vi "Check Configs Exist.vi"(8 "error in (no error)":errorcluster, 11 "picoG in":refnum<class "picoG.lvclass">) -> (0 "error out":errorcluster, 3 "picoG out":refnum<class "picoG.lvclass">)   [LabVIEW 2020, in "PicoG-App.lvlib" / "picoG.lvclass"]
uses:
  picoG.lvclass
  PicoG-App.lvlib
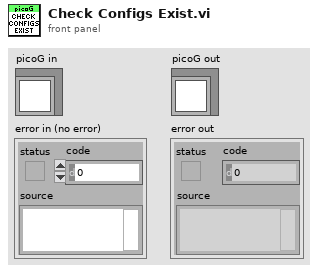
[diagram p1: front panel]
types:
  T1 = typedef "PicoG-App.lvlib/Paths.ctl" = cluster{"User picoG":path, "System picoG":path, "User Config":path, "System Config":path}
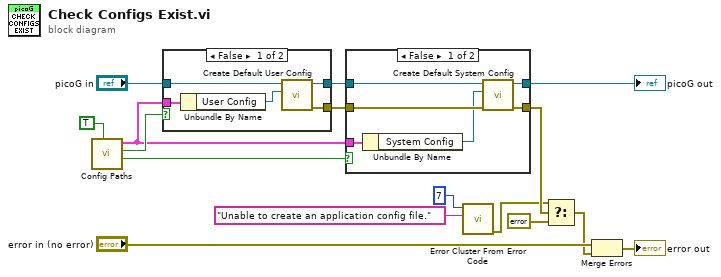
[diagram p0: block diagram]
diagram:
  n1 = call "Config Paths.vi"("Create if Missing? (F)"=TRUE ("Create if Missing? (T)")) -> ("System Config Exists"=w10:bool, "User Config Exists"=w14:bool, "Paths"=w11:T1)  [unwired: 7 in, 1 out]
  n2 = case shown="False" w14 {
    tunnel: "picoG in" -> [w20 w22]
    tunnel: w11 -> [w21 _]
    tunnel: [w18 w22] -> w12
    tunnel: [w17 _] -> w9
    frame False {
      n3 = Unbundle By Name(w21) -> ("User Config"=w19:path)
      n4 = call "Create Default User Config.vi"("User Config Path"=w19, "App in"=w20) -> ("error out"=w17:errorcluster, "App out"=w18:refnum<class "picoG.lvclass">)  [unwired: 8 in]
    }
    frame True {
    }
  }
  n5 = case shown="False" w10 {
    tunnel: w12 -> [w27 w30]
    tunnel: w11 -> [w28 _]
    tunnel: [w23 w30] -> w1
    tunnel: [w24 w29] -> w8
    tunnel: w9 -> [w26 w29]
    frame False {
      n6 = Unbundle By Name(w28) -> ("System Config"=w25:path)
      n7 = call "Create Default System Config.vi"("error in (no error)"=w26, "System Config Path"=w25, "App in"=w27) -> ("error out"=w24:errorcluster, "App out"=w23:refnum<class "picoG.lvclass">)  [unwired: 7 in]
    }
    frame True {
    }
  }
  "picoG out" <- w1
  n8 = call <vilib>:"Error Cluster From Error Code.vi"("error message (\"\")"="Unable to create an application config file." ("error message (\"\")"), "error code (0)"=7) -> ("error out"=w5:errorcluster)  [unwired: 7 in]
  n9 = Select(t=w5, s=w8, f=errorcluster {"status"=FALSE, "code"=0, "source"=""}) -> (s? t:f=w2:errorcluster)
  n10 = Merge Errors("error in (no error)", w2) -> (→"error out":errorcluster)
